vi "Check Solution Exists.vi"() -> ()   [LabVIEW 2020]
panel:
  out "Error Out":errorcluster
  in  "Error In":errorcluster
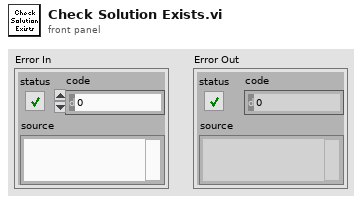
[diagram p1: front panel]
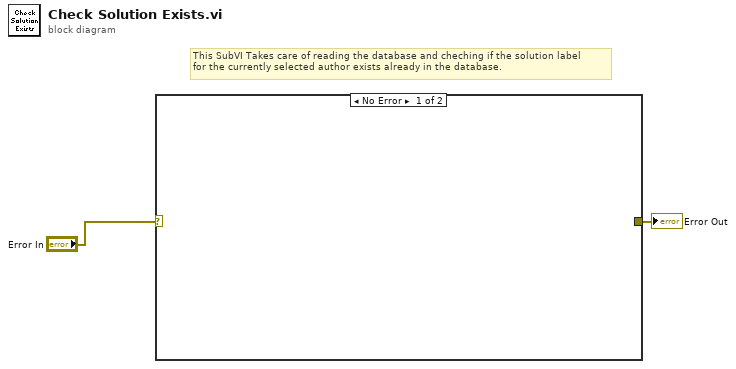
[diagram p0: block diagram]
diagram:
  # "This SubVI Takes care of reading the database and cheching if the solution label\nfor the currently selected author exists already in the database."
  n1 = case shown="No Error" "Error In" {
    selector: "Error In" -> [_ w3]
    tunnel: [_ w3] -> w1
    frame No Error {
    }
    frame Error {
    }
  }
  "Error Out" <- w1
